vi "Setup Timer 2.vi"(7 "Next State":string, 8 "error in (no error)":errorcluster, 9 "Count":i32, 10 "Period":i32, 11 "Timer On":bool) -> (0 "error out":errorcluster)   [LabVIEW 2015, in "Tool Module.lvlib"]
doc: "Start/Stop and specify the timing period and number of time periods (Count) for Timer 2.\n_____\nCreated using Delacor QMH Event Scripter 4.2.1.88."
uses:
  Tool Module.lvlib
  Setup Timer 2 Argument--cluster.ctl
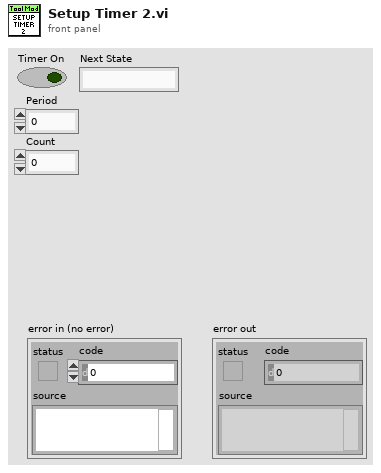
[diagram p1: front panel]
types:
  T1 = typedef "Tool Module.lvlib/Setup Timer 2 Argument--cluster.ctl" = cluster{"Timer On":bool, "Period":i32, "Count":i32, "Next State":string}
  T2 = typedef "Tool Module.lvlib/Request Events--cluster.ctl" = cluster{"Stop Module":refnum<user-event>, "Show Panel":refnum<user-event>, "Hide Panel":refnum<user-event>, "Get Module Execution Status":refnum<user-event>, "Show Diagram":refnum<user-event>, "Test Trig 2":refnum<user-event>, "GOTO":refnum<user-event>, "Start Inspect":refnum<user-event>, "CONNECT":refnum<user-event>, "Get All Inspect Data":refnum<user-event>, "Get Inspection Limits":refnum<user-event>, "Set Inspection Limits":refnum<user-event>, "Update Motion Status":refnum<user-event>, "Start Data Monitor":refnum<user-event>, "Get FPGA Setup Params":refnum<user-event>, "Set FPGA Setup Params":refnum<user-event>, "Set Tool Config":refnum<user-event>, "Get Tool Config":refnum<user-event>, "Set Integration Count":refnum<user-event>, "Set Laser Params":refnum<user-event>, "Get Mtrl Ctrl Reg":refnum<user-event>, "Commit Ctrl Reg":refnum<user-event>, "Set Event Logger":refnum<user-event>, "Write to File":refnum<user-event>, "Read from File":refnum<user-event>, "Set Device Temp Thresholds":refnum<user-event>, "Get Cycle Count":refnum<user-event>, "Return FPGA Setup Data":refnum<user-event>, "Update FPGA Setup Data":refnum<user-event>, "Setup Timer 1":refnum<user-event>, "Setup Timer 2":refnum<user-event>}
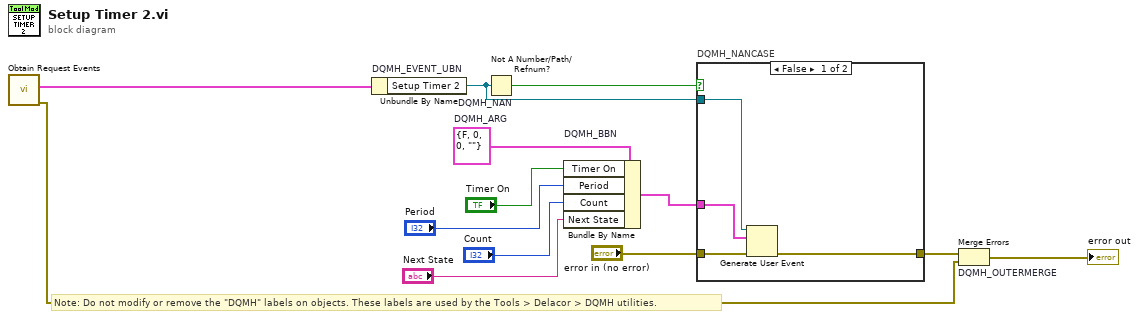
[diagram p0: block diagram]
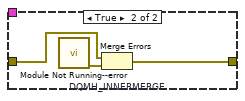
[diagram p2: hidden frame]
diagram:
  w7 = T1 {"Timer On"=FALSE, "Period"=0, "Count"=0, "Next State"=""}  # DQMH_ARG
  # "Note: Do not modify or remove the \"DQMH\" labels on objects. These labels are used by the Tools > Delacor > DQMH utilities."
  n1 = call "Obtain Request Events.vi"() -> ("error out"=w6:errorcluster, "Tool Module Request Events"=w5:T2)  [unwired: 10 in]
  n2 = Unbundle By Name "DQMH_EVENT_UBN"(w5) -> ("Setup Timer 2"=w9:refnum<user-event>)
  n3 = Not A Number/Path/Refnum? "DQMH_NAN"(number/path/refnum=w9) -> (NaN/Path/Refnum?=w10:bool)
  n4 = Bundle By Name "DQMH_BBN"(cluster=w7, "Timer On"="Timer On", "Period"="Period", "Count"="Count", "Next State"="Next State") -> (w11:T1)
  n5 = case "DQMH_NANCASE" shown="False" w10 {
    tunnel: "error in (no error)" -> [w17 w20]
    tunnel: [w16 w19] -> w8
    tunnel: w9 -> [w15 _]
    tunnel: w11 -> [w14 _]
    frame False {
      n6 = Generate User Event(user event=w15, event data cluster=w14, error in=w17) -> (error out=w16:errorcluster)  [unwired: 1 in, 1 out]
    }
    frame True {
      n7 = call "Module Not Running--error.vi"() -> ("error out"=w18:errorcluster)  [unwired: 11 in]
      n8 = Merge Errors "DQMH_INNERMERGE"(w20, w18) -> (w19:errorcluster)
    }
  }
  n9 = Merge Errors "DQMH_OUTERMERGE"(w8, w6) -> (→"error out":errorcluster)
